vi "单点数据解析.vi"(4 "字符串":string) -> (1 "*(类型 *) &x":i32)   [LabVIEW 2024]
panel:
  out "连接的字符串":string
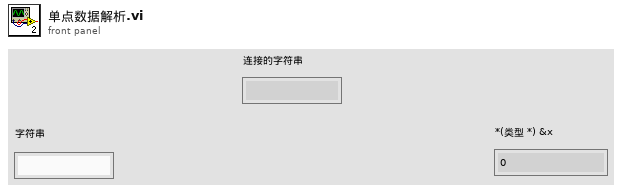
[diagram p1: front panel]
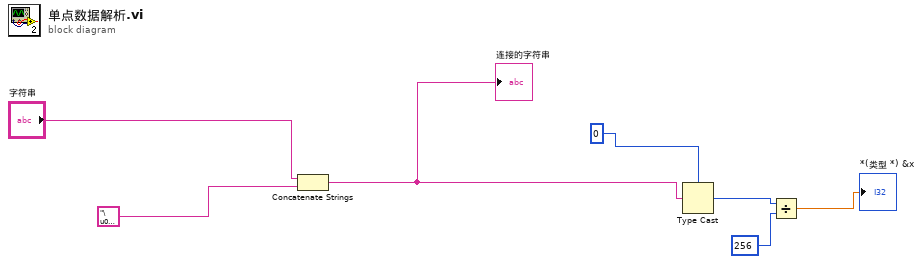
[diagram p0: block diagram]
diagram:
  n1 = Concatenate Strings("字符串", "\u0000" ("字符串")) -> (w5:string)
  "连接的字符串" <- w5
  n2 = Type Cast(type=0, x=w5) -> (*(type *) &x=w3:i32)
  n3 = Divide(x=w3, y=256) -> (x/y=→"*(类型 *) &x":dbl)
